vi "Keithley 2400 Settings.vi"(8 "error in (no error)":errorcluster, 10 "Keithley 2400 Setting String":string[](array[string]), 11 "Keithley 2400 Visa Resource":refnum<visa-resource-name>) -> (0 "error out":errorcluster)   [LabVIEW 2019]
panel:
  # "This VI reads the input settings and updates\nthem for the Keithley 2400\n\nJustin Young\n2012.06.23"
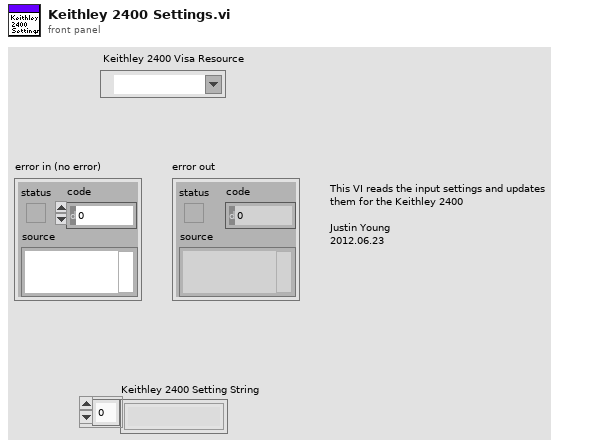
[diagram p1: front panel]
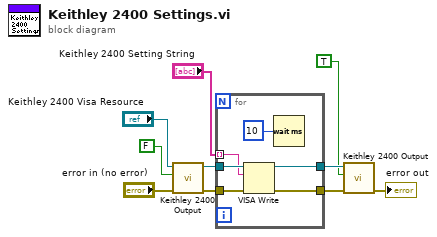
[diagram p0: block diagram]
diagram:
  n1 = call "Keithley 2400 Output.vi"("error in (no error)"="error in (no error)", "Enable Output (T: Enable)"=FALSE, "VISA resource name"="Keithley 2400 Visa Resource") -> ("error out"=w9:errorcluster, "VISA resource name out"=w8:refnum<visa-resource-name>)  [unwired: 7 in]
  n2 = for {
    tunnel: w8 -> [w16]
    tunnel: w9 -> [w15]
    tunnel: [w14] -> w7
    tunnel: [w13] -> w6
    tunnel: "Keithley 2400 Setting String" -> [w12] mode=indexing
    n3 = VISA Write(VISA resource name=w16, write buffer=w12, error in (no error)=w15) -> (VISA resource name out=w13:refnum<visa-resource-name>, error out=w14:errorcluster)  [unwired: 1 out]
    n4 = Wait (ms)(milliseconds to wait=u32 10) -> ()  [unwired: 1 out]
  }
  n5 = call "Keithley 2400 Output.vi"("error in (no error)"=w7, "Enable Output (T: Enable)"=TRUE, "VISA resource name"=w6) -> ("error out"=→"error out":errorcluster)  [unwired: 7 in, 1 out]
